vi "checkOverheat.vi"(8 "error in (no error)":errorcluster, 11 "Thermocouple in":refnum<class "Thermocouple.lvclass">) -> (0 "error out":errorcluster, 2 "overtempIsTrue":bool, 3 "Thermocouple out":refnum<class "Thermocouple.lvclass">)   [LabVIEW 2013, in "Thermocouple.lvclass"]
uses:
  Thermocouple.lvclass
  Thermocouple.lvclass/Thermocouple.ctl
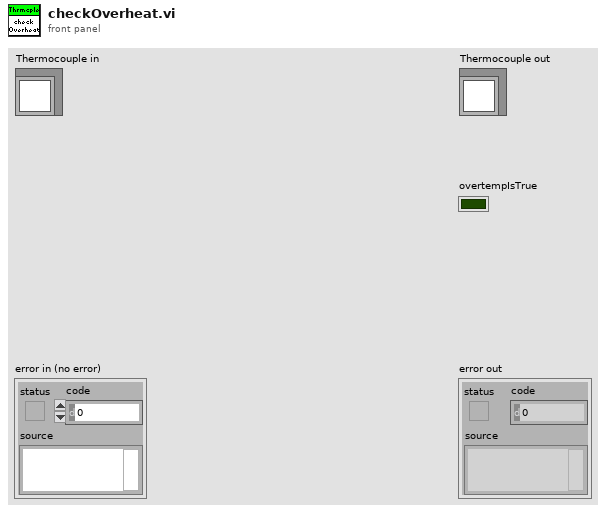
[diagram p1: front panel]
types:
  T1 = typedef "MotorOverheatTemperature.ctl" = dbl[unit]
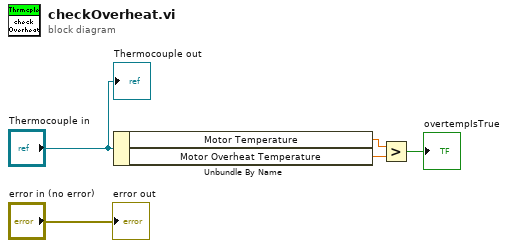
[diagram p0: block diagram]
diagram:
  n1 = Unbundle By Name("Thermocouple in") -> ("Motor Temperature"=w1:dbl[unit], "Motor Overheat Temperature"=w3:T1)
  n2 = Greater?(x=w1, y=w3) -> (0:→"overtempIsTrue":bool)
  "error out" <- "error in (no error)"
  "Thermocouple out" <- "Thermocouple in"
